vi "find_scope_data_Q_errors.vi"(7 "scope Q data":T1) -> (8 "scope Q data 2":T1, 13 "Error?":bool)   [LabVIEW 2023]
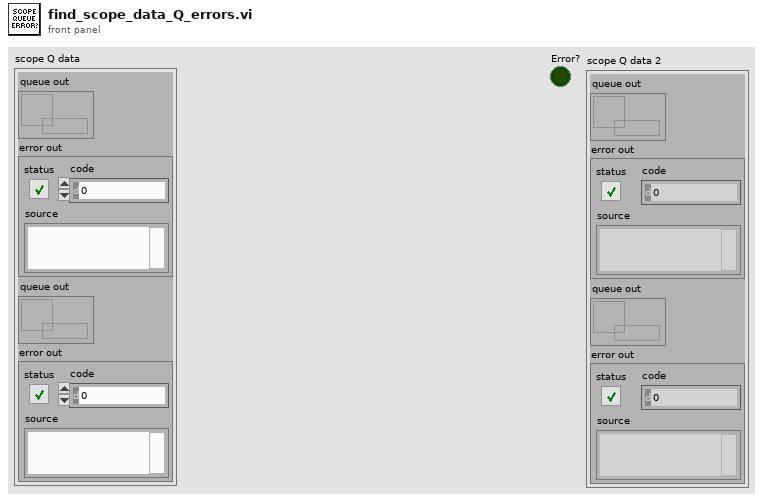
[diagram p1: front panel]
types:
  T1 = cluster{"queue out":refnum<queue>, "error out":errorcluster, "queue out":refnum<queue>, "error out":errorcluster}
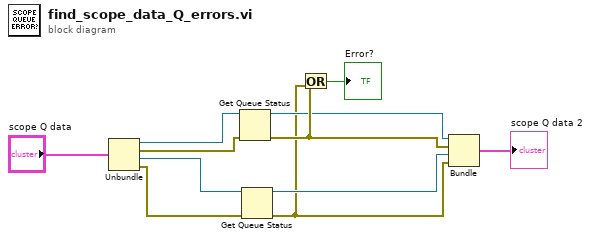
[diagram p0: block diagram]
diagram:
  n1 = Unbundle("scope Q data") -> ("queue out"=w7:refnum<queue>, "error out"=w6:errorcluster, "queue out"=w5:refnum<queue>, "error out"=w4:errorcluster)
  n2 = Get Queue Status(queue=w7, error in (no error)=w6) -> (queue out=w10:refnum<queue>, error out=w11:errorcluster)  [unwired: 1 in, 6 out]
  n3 = Get Queue Status(queue=w5, error in (no error)=w4) -> (queue out=w9:refnum<queue>, error out=w8:errorcluster)  [unwired: 1 in, 6 out]
  n4 = Or(x=w11, y=w8) -> (x .or. y?=→"Error?":bool)
  n5 = Bundle("queue out"=w10, "error out"=w11, "queue out"=w9, "error out"=w8) -> (→"scope Q data 2":T1)  [unwired: 1 in]
